vi "tituloDoArquivo.vi"(6 "area":dbl caption="Área da célula", 8 "temperatura":dbl caption="Temperatura da célula", 9 "Tipo":string caption="Tipo da célula", 10 "Nome da célula":string, 11 "file path (dialog if empty)":path) -> ()   [LabVIEW 2012]
uses:
  <vilib>/Utility/file.llb/Write To Spreadsheet File (string).vi
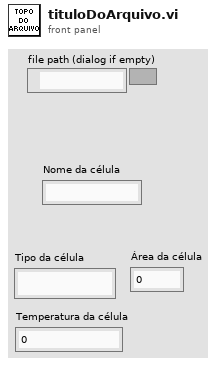
[diagram p1: front panel]
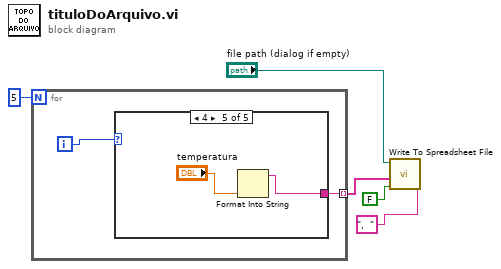
[diagram p0: block diagram]
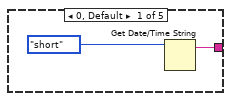
[diagram p2: hidden frame]
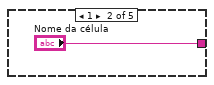
[diagram p3: hidden frame]
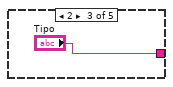
[diagram p4: hidden frame]
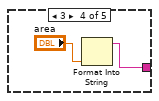
[diagram p5: hidden frame]
diagram:
  n1 = for {
    N: 5 -> [_]
    tunnel: [w7] -> w5 mode=indexing
    i -> [w6]
    n2 = case shown="4" w6 {
      tunnel: [w9 "Nome da célula" "Tipo" w12 w14] -> w7
      frame 0, Default {
        n3 = Get Date/Time String(date format (0)=enum16{"short", "long", "abbreviated"}."short") -> (date string=w9:string)  [unwired: 2 in, 1 out]
      }
      frame 1 {
      }
      frame 2 {
      }
      frame 3 {
        n4 = Format Into String("area") -> (resulting string=w12:string)  [unwired: 3 in, 1 out]
      }
      frame 4 {
        n5 = Format Into String("temperatura") -> (resulting string=w14:string)  [unwired: 3 in, 1 out]
      }
    }
  }
  n6 = call-poly <vilib>:"Write To Spreadsheet File.vi"("delimiter (\\t)"=",  " ("delimiter (\\t)"), "append to file? (new file:F)"=FALSE, "1D data"=w5, "file path (dialog if empty)"="file path (dialog if empty)") -> ()  [unwired: 4 in, 1 out]
